vi "hysteresis_PI_no_sat.vi"(7 "N_hyst":i32, 8 "y_vec_in":sgl[](array[numeric])=[0.0, 0.0, 0.0, 0.0, 0.0, 0.0, 0.0], 9 "r_s":sgl[](array[numeric])=[0.0, 0.0, 0.0, 0.0, 0.0, 0.0, 0.0], 10 "w_s":sgl[](array[numeric])=[0.0, 0.0, 0.0, 0.0, 0.0, 0.0, 0.0], 11 "uk":sgl format="%#_13g") -> (0 "y_vec_out":sgl[](array[numeric]), 3 "H_of_ik":sgl)   [LabVIEW 2017]
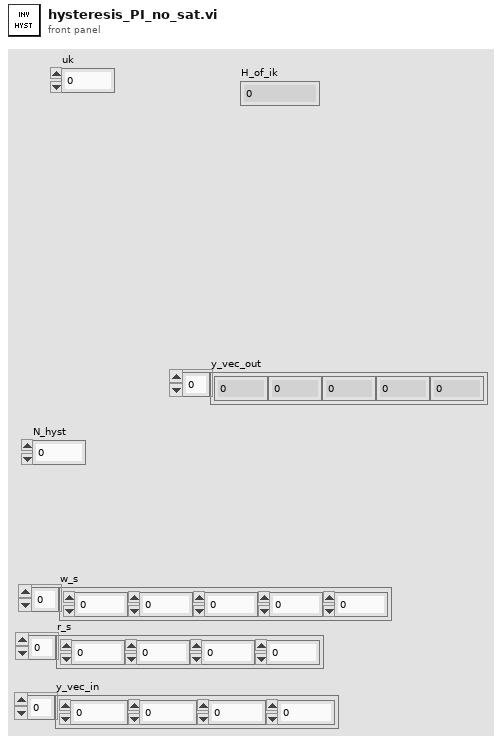
[diagram p1: front panel]
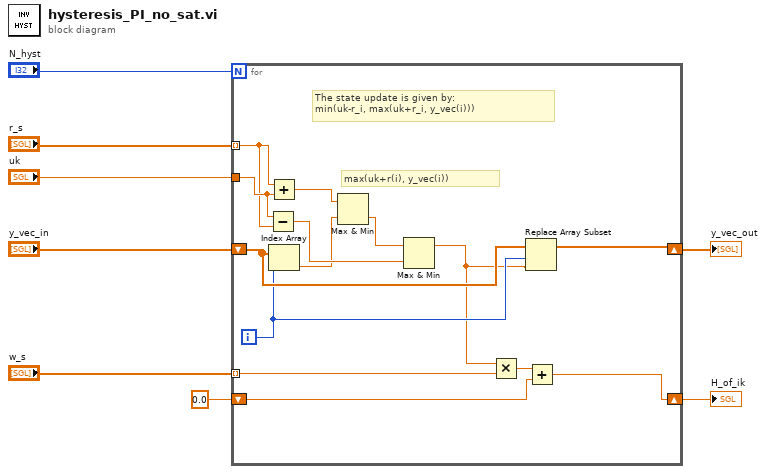
[diagram p0: block diagram]
diagram:
  n1 = for {
    N: "N_hyst" -> [_]
    tunnel: "w_s" -> [w17] mode=indexing
    tunnel: "r_s" -> [w20] mode=indexing
    shift-right: [w14] -> w8
    shift-left: sgl 0.0 -> [w15]
    tunnel: "uk" -> [w21]
    shift-right: [w13] -> w4
    shift-left: "y_vec_in" -> [w12]
    i -> [w11]
    # "max(uk+r(i), y_vec(i))"
    # "The state update is given by:\nmin(uk-r_i, max(uk+r_i, y_vec(i)))"
    n2 = Subtract(x=w21, y=w20) -> (x-y=w19:sgl)
    n3 = Add(x=w20, y=w21) -> (x+y=w22:sgl)
    n4 = Index Array(array=w12, index=w11) -> (element=w18:sgl)
    n5 = Max & Min(x=w22, y=w18) -> (min(x,y)=w10:sgl)  [unwired: 1 out]
    n6 = Max & Min(x=w10, y=w19) -> (max(x,y)=w9:sgl)  [unwired: 1 out]
    n7 = Multiply(x=w9, y=w17) -> (x*y=w16:sgl)
    n8 = Replace Array Subset(array=w12, new element=w9, index=w11) -> (w13:sgl[])
    n9 = Add(x=w16, y=w15) -> (x+y=w14:sgl)
  }
  "H_of_ik" <- w8
  "y_vec_out" <- w4
